vi "LED-Facade.vi"(9 "Container State":T3, 10 "Display State In":T2, 11 "Data In":T4) -> (0 "Action":T1, 1 "Display State Out":T2, 3 "Data Out":T4)   [LabVIEW 2012, in "LED Display.xctl"]
doc: "This is the Façade of the XControl. The Façade VI manages the different states the XControl can get into and how it responds to user events. Hence this is a giant event handler VI that is called by LabVIEW only when there is an event pending for it to handle. Whenever the Façade is called, LabVIEW passes in the current data and state of the XControl as inputs. The Façade VI then handles the event and updates the data and state and returns them to LabVIEW to be stored with the control."
uses:
  LED Display.xctl
  LED-Data.ctl
  <vilib>/_xctls/Container State.ctl
  LED-State.ctl
  <vilib>/_xctls/Action.ctl
  <vilib>/_xctls/XControlSupport.lvlib
panel:
  out "LED Display":bool[][](array[boolean])
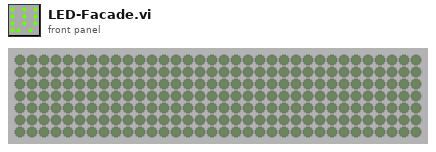
[diagram p1: front panel]
types:
  T1 = typedef "XControlSupport.lvlib/Action.ctl" = cluster{"Data Changed?":bool, "State Changed?":bool, "Action Name":string}
  T2 = typedef "LED Display.xctl/LED-State.ctl" = cluster{"Flags":u64}
  T3 = typedef "XControlSupport.lvlib/Container State.ctl" = cluster{"Indicator?":bool, "Run Mode?":bool, " Refnum":refnum<vi>}
  T4 = typedef "LED Display.xctl/LED-Data.ctl" = string
  T5 = typedef "LVRectTypeDef.ctl" = cluster{"Left":i16, "Top":i16, "Right":i16, "Bottom":i16}
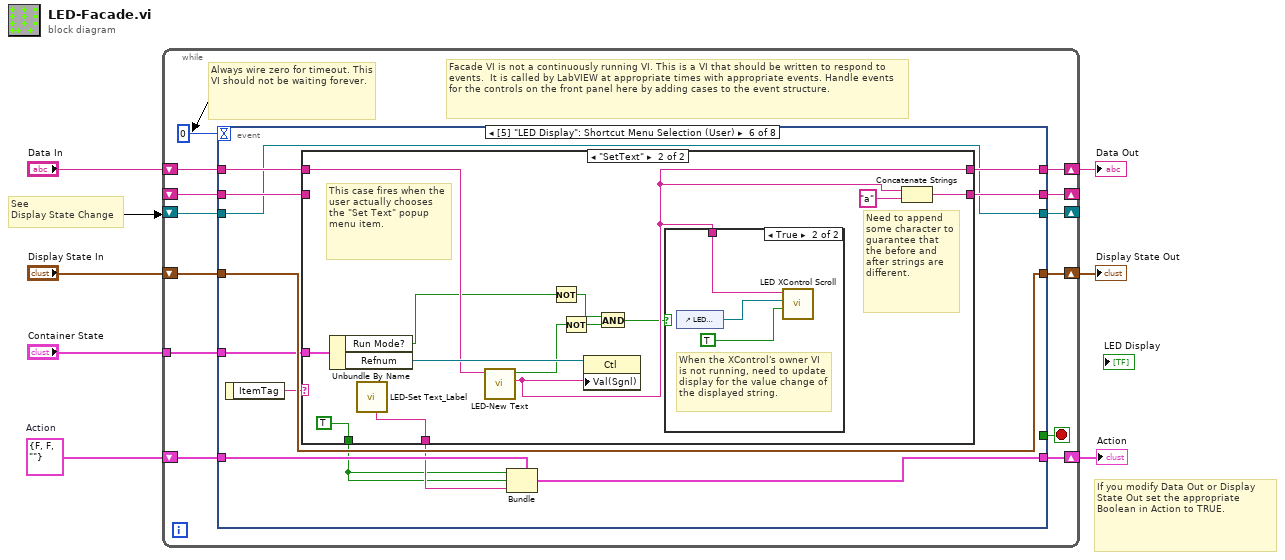
[diagram p0: block diagram]
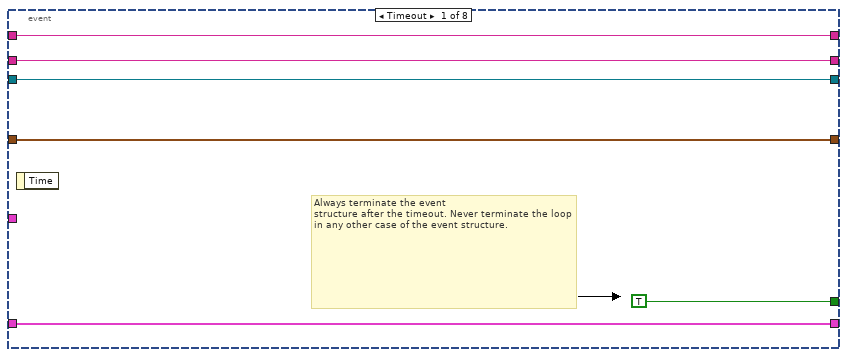
[diagram p2: hidden frame]
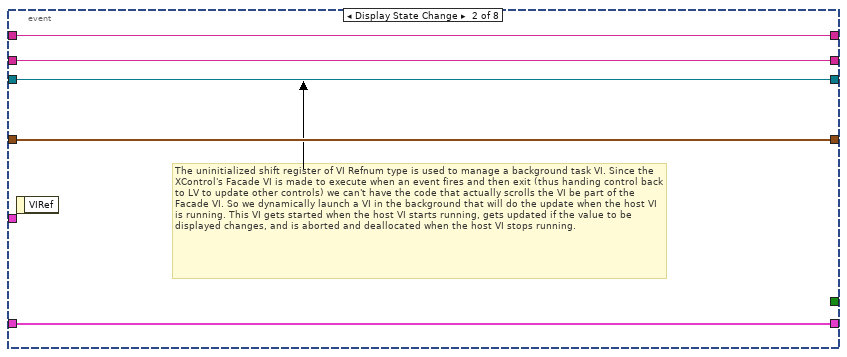
[diagram p3: hidden frame]
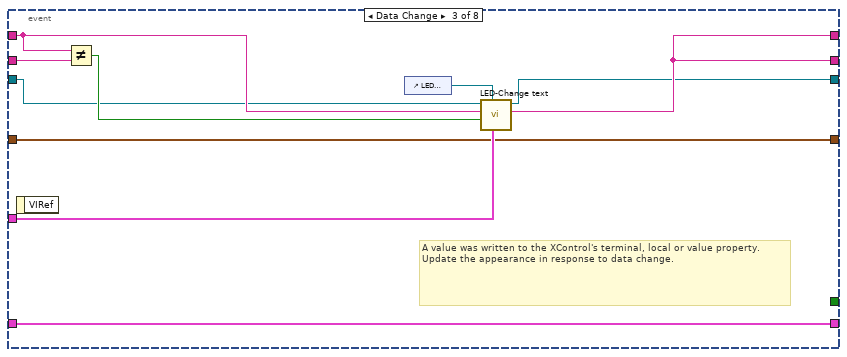
[diagram p4: hidden frame]
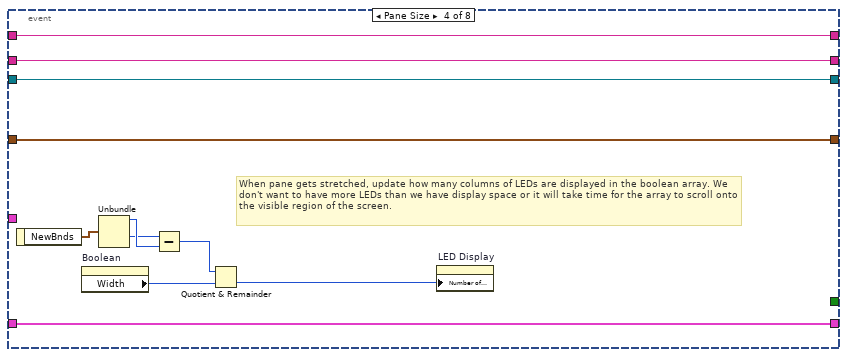
[diagram p5: hidden frame]
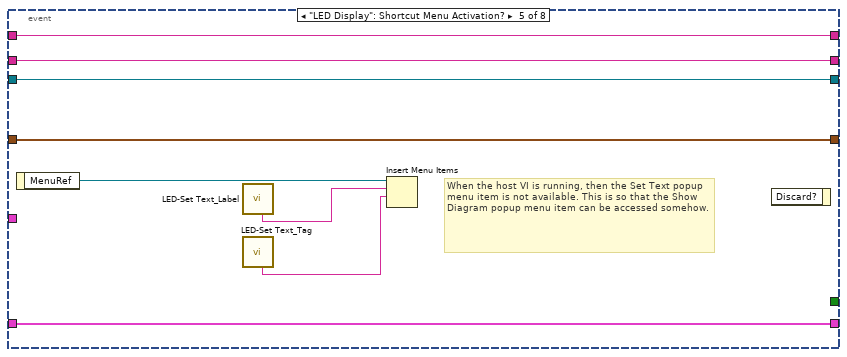
[diagram p6: hidden frame]
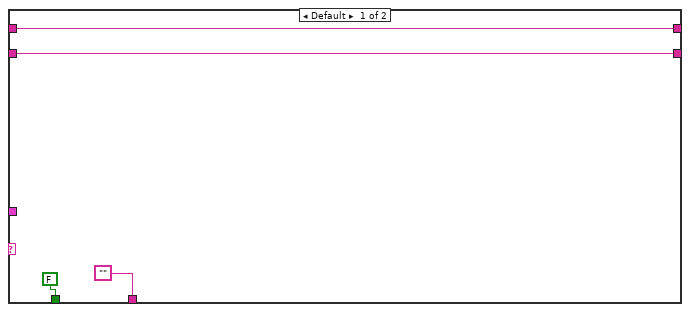
[diagram p7: hidden frame]
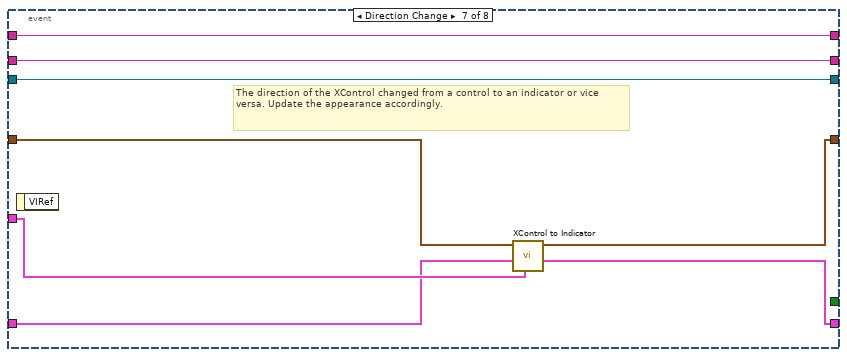
[diagram p9: hidden frame]
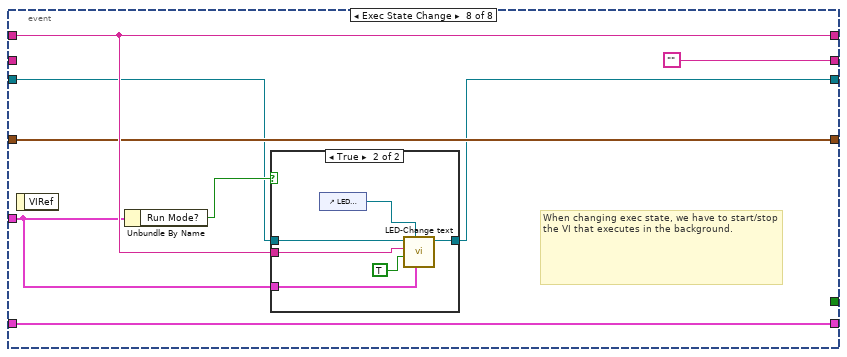
[diagram p10: hidden frame]
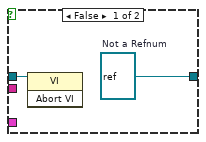
[diagram p11: hidden frame]
diagram:
  w1 = T1 {"Data Changed?"=FALSE, "State Changed?"=FALSE, "Action Name"=""}  # Action
  # "See\nDisplay State Change"
  # "If you modify Data Out or Display State Out set the appropriate Boolean in Action to TRUE."
  n1 = while {
    shift-right: [w19] -> w4
    shift-left: "Display State In" -> [w20]
    tunnel: "Container State" -> [w16]
    shift-right: [w14] -> w7
    shift-left: "Data In" -> [w15]
    shift-right: [w12] -> w2
    shift-left: w1 -> [w13]
    shift-right: [w11] -> _
    shift-left: _ -> [w10]
    shift-right: [w9] -> _
    shift-left: _ -> [w8]
    stop <- w18 stop-if-true
    # "Facade VI is not a continuously running VI. This is a VI that should be written to respond to events.  It is called by LabVIEW at appropriate times with appropriate events. Handle events for the controls on the front panel here by adding cases to the event structure."
    # "Always wire zero for timeout. This\nVI should not be waiting forever."
    n2 = event shown="[5] \"LED Display\": Shortcut Menu Selection (User)" {
      selector: _ -> [_ _ _ _ _ _ _ _]
      dyn-events: _ -> [_ _ _ _ _ _ _ _]
      timeout: 0 -> [_ _ _ _ _ _ _ _]
      tunnel: w20 -> [w24 w31 w32 w50 w59 w70 w97 w103]
      tunnel: [w24 w31 w32 w50 w59 w70 w96 w103] -> w19
      tunnel: [TRUE _ _ _ _ _ _ _] -> w18
      tunnel: w16 -> [_ _ w41 _ _ w62 w99 w105]
      tunnel: w15 -> [w23 w29 w36 w52 w57 w66 w100 w106]
      tunnel: [w23 w29 w37 w52 w57 w68 w100 w106] -> w14
      tunnel: [w25 w30 w35 w49 w56 w71 w94 w104] -> w12
      tunnel: w13 -> [w25 w30 w35 w49 w56 w72 w95 w104]
      tunnel: [w22 w28 w37 w51 w58 w69 w98 ""] -> w11
      tunnel: w10 -> [w22 w28 w40 w51 w58 w65 w98 _]
      tunnel: [w21 w27 w34 w44 w55 w61 w93 w102] -> w9
      tunnel: w8 -> [w21 w27 w33 w44 w55 w61 w93 w101]
      event Timeout {
        # "Always terminate the event\nstructure after the timeout. Never terminate the loop in any other case of the event structure."
        n3 = event-data() -> ()  [unwired: 1 in, 1 out]
      }
      event Display State Change {
        # "The uninitialized shift register of VI Refnum type is used to manage a background task VI. Since the XControl's Facade VI is made to execute when an event fires and then exit (thus handing control back to LV to update other controls) we can't have the code that actually scrolls the VI be part of the Facade VI. So we dynamically launch a VI in the background that will do the update when the host VI is running. This VI gets started when the host VI starts running, gets updated if the value to be displayed changes, and is aborted and deallocated when the host VI stops running."
        n4 = event-data() -> ()  [unwired: 1 in, 1 out]
      }
      event Data Change {
        # "A value was written to the XControl's terminal, local or value property.\nUpdate the appearance in response to data change."
        n5 = event-data() -> ()  [unwired: 1 in, 1 out]
        n6 = Not Equal?(x=w36, y=w40) -> (x != y?=w39:bool)
        n7 = control-ref of="LED Display"() -> (w38:refnum<vi>)
        n8 = call "LED-Change text.vi"("Container State"=w41, "LED Display"=w38, "Should Change?"=w39, "Data In"=w36, "vi reference in"=w33) -> ("Data Out"=w37:T4, "vi reference out"=w34:refnum<vi>)  [unwired: 4 in, 1 out]
      }
      event Pane Size {
        # "When pane gets stretched, update how many columns of LEDs are displayed in the boolean array. We don't want to have more LEDs than we have display space or it will take time for the array to scroll onto the visible region of the screen."
        n9 = event-data() -> ("NewBnds"=w48:T5)  [unwired: 1 in]
        n10 = property on="Boolean" class="Bool (strict)"() -> ("Width"=w42:u32)  [unwired: 2 in, 2 out]
        n11 = Unbundle(w48) -> ("Left"=w46:i16, "Right"=w45:i16)  [unwired: 2 out]
        n12 = Subtract(x=w45, y=w46) -> (x-y=w47:i16)
        n13 = Quotient & Remainder(x=w47, y=w42) -> (floor(x/y)=w43:u32)  [unwired: 1 out]
        n14 = property on="LED Display" class="Arr (strict)"("Number of Columns"=w43) -> ()  [unwired: 2 in, 2 out]
      }
      event "LED Display": Shortcut Menu Activation? {
        # "When the host VI is running, then the Set Text popup menu item is not available. This is so that the Show Diagram popup menu item can be accessed somehow."
        n15 = event-data() -> ("MenuRef"=w60:refnum<k9>)  [unwired: 1 in]
        n16 = call "LED-Set Text_Label.vi"() -> ("\"Set Text\" Label"=w54:string)  [unwired: 11 in]
        n17 = call "LED-Set Text_Tag.vi"() -> ("\"Set Text\" Label"=w53:string)  [unwired: 11 in]
        n18 = Insert Menu Items(7:w53, 8:w54, 9:w60) -> ()  [unwired: 3 in, 3 out]
        n19 = event-data() -> ()  [unwired: 2 in, 1 out]
      }
      event "LED Display": Shortcut Menu Selection (User) {
        n20 = event-data() -> ("ItemTag"=w67:string)  [unwired: 1 in]
        n21 = case shown="\"SetText\"" w67 {
          tunnel: [w75 w88] -> w69
          tunnel: [w76 w82] -> w68
          tunnel: [FALSE TRUE] -> w63
          tunnel: w66 -> [w76 w83]
          tunnel: w65 -> [w75 _]
          tunnel: ["" w86] -> w64
          tunnel: w62 -> [_ w85]
          frame Default {
          }
          frame "SetText" {
            # "This case fires when the user actually chooses the \"Set Text\" popup menu item."
            # "Need to append some character to guarantee that the before and after strings are different."
            n22 = Unbundle By Name(w85) -> ("Run Mode?"=w81:bool, "Refnum"=w84:refnum<vi>)
            n23 = call "LED-Set Text_Label.vi"() -> ("\"Set Text\" Label"=w86:string)  [unwired: 11 in]
            n24 = call "LED-New Text.vi"("Current Text"=w83) -> ("New text"=w82:string, "Cancelled?"=w78:bool)  [unwired: 9 in]
            n25 = Not(x=w81) -> (.not. x?=w80:bool)
            n26 = Not(x=w78) -> (.not. x?=w79:bool)
            n27 = property class="Ctl"(reference=w84, "Val(Sgnl)"=w82) -> ()  [unwired: 1 in, 2 out]
            n28 = And(x=w80, y=w79) -> (x .and. y?=w77:bool)
            n29 = case shown="True" w77 {
              tunnel: w82 -> [_ w92]
              frame False {
              }
              frame True {
                # "When the XControl's owner VI\nis not running, need to update\ndisplay for the value change of\nthe displayed string."
                n30 = control-ref of="LED Display"() -> (w91:refnum<vi>)
                n31 = call "LED XControl Scroll.vi"("Single pass?"=TRUE, "LEDDisplay"=w91, "String"=w92) -> ()  [unwired: 9 in]
              }
            }
            n32 = Concatenate Strings(w82, "a" ("string")) -> (w88:string)
          }
        }
        n33 = Bundle(cluster=w72, "Data Changed?"=w63, "State Changed?"=w63, "Action Name"=w64) -> (w71:T1)
      }
      event Direction Change {
        # "The direction of the XControl changed from a control to an indicator or vice versa. Update the appearance accordingly."
        n34 = event-data() -> ()  [unwired: 1 in, 1 out]
        n35 = call "XControl to Indicator.vi"("Container State"=w99, "Action In"=w95, "Display State In"=w97) -> ("Action Out"=w94:T1, "Display State Out"=w96:T2)  [unwired: 7 in]
      }
      event Exec State Change {
        # "When changing exec state, we have to start/stop the VI that executes in the background."
        n36 = event-data() -> ()  [unwired: 1 in, 1 out]
        n37 = Unbundle By Name(w105) -> ("Run Mode?"=w108:bool)
        n38 = case shown="True" w108 {
          tunnel: [w110 w112] -> w102
          tunnel: w106 -> [_ w116]
          tunnel: w105 -> [_ w114]
          tunnel: w101 -> [w109 w111]
          frame False {
            w110 = refnum<vi> refnum  # Not a Refnum
            n39 = invoke class="VI" method="Abort VI"(reference=w109) -> ()  [unwired: 2 in, 3 out]
          }
          frame True {
            n40 = control-ref of="LED Display"() -> (w113:refnum<vi>)
            n41 = call "LED-Change text.vi"("Container State"=w114, "LED Display"=w113, "Should Change?"=TRUE, "Data In"=w116, "vi reference in"=w111) -> ("vi reference out"=w112:refnum<vi>)  [unwired: 4 in, 2 out]
          }
        }
      }
    }
  }
  "Display State Out" <- w4
  "Data Out" <- w7
  "Action" <- w2
